vi "Configure Trigger Mode.vi"(8 "error in (no error)":errorcluster, 10 "Trigger Mode":T1, 11 "DG645 in":refnum<class "DG645.lvclass">) -> (0 "error out":errorcluster, 3 "DG645 out":refnum<class "DG645.lvclass">)   [LabVIEW 2018, in "DG645.lvlib" / "DG645.lvclass"]
uses:
  DG645.lvclass
  PPLs/Digital Delay Generator/Parent/Digital Delay Generator.lvlibp/Custom Controls/Trigger Mode.ctl
  DG645.lvclass/DG645.ctl
  <instrlib>/Stanford Research DG645/Stanford Research DG645.lvlib
  PPLs/Digital Delay Generator/Parent/Digital Delay Generator.lvlibp/Digital Delay Generator.lvclass
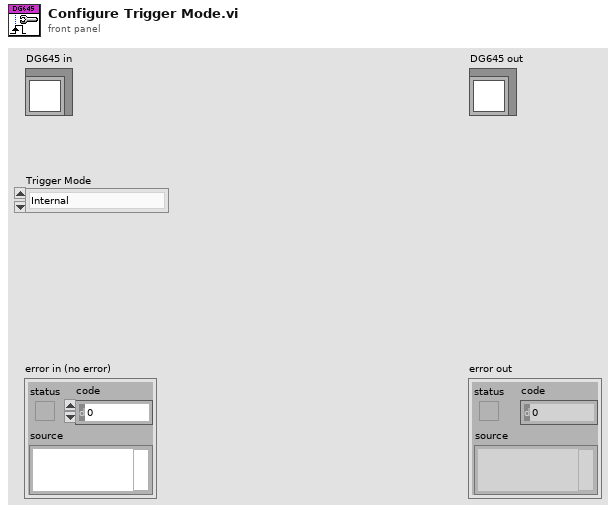
[diagram p1: front panel]
types:
  T1 = typedef "Digital Delay Generator.lvlibp/Digital Delay Generator.lvclass/Trigger Mode.ctl" = enum16{"Internal", "External Rising Edge", "External Falling Edge", "Single Shot Internal Rising Edge", "Single Shot External Rising Edge", "Single Shot", "Line"}
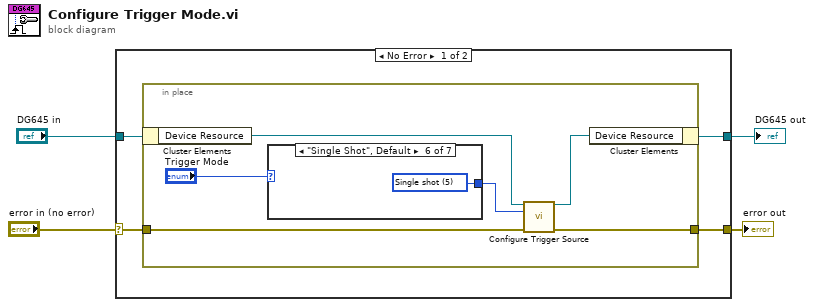
[diagram p0: block diagram]
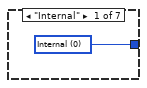
[diagram p2: hidden frame]
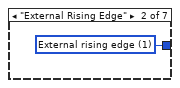
[diagram p3: hidden frame]
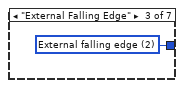
[diagram p4: hidden frame]
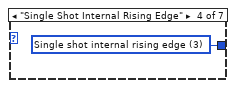
[diagram p5: hidden frame]
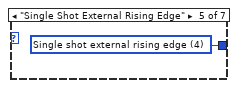
[diagram p6: hidden frame]
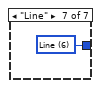
[diagram p7: hidden frame]
diagram:
  n1 = case shown="No Error" "error in (no error)" {
    selector: "error in (no error)" -> [w7 w23]
    tunnel: [w6 w23] -> w3
    tunnel: [w5 w22] -> w2
    tunnel: "DG645 in" -> [w8 w22]
    frame No Error {
      n2 = in-place {
        in-place-border: w7 -> [w13]
        in-place-border: [w12] -> w6
        n3 = in-place-cluster #1(w8) -> ("Device Resource"=w14:refnum<visa-resource-name>)
        n4 = case shown="\"Single Shot\", Default" "Trigger Mode" {
          tunnel: [w15 w16 w17 w18 w19 w20 w21] -> w10
          frame "Internal" {
            w15 = u16 0 items=["Internal", "External rising edge", "External falling edge", "Single shot internal rising edge", "Single shot external rising edge", "Single shot", "Line"] ("Trigger Source (5:Single Shot)")
          }
          frame "External Rising Edge" {
            w16 = u16 1 items=["Internal", "External rising edge", "External falling edge", "Single shot internal rising edge", "Single shot external rising edge", "Single shot", "Line"] ("Trigger Source (5:Single Shot)")
          }
          frame "External Falling Edge" {
            w17 = u16 2 items=["Internal", "External rising edge", "External falling edge", "Single shot internal rising edge", "Single shot external rising edge", "Single shot", "Line"] ("Trigger Source (5:Single Shot)")
          }
          frame "Single Shot Internal Rising Edge" {
            w18 = u16 3 items=["Internal", "External rising edge", "External falling edge", "Single shot internal rising edge", "Single shot external rising edge", "Single shot", "Line"] ("Trigger Source (5:Single Shot)")
          }
          frame "Single Shot External Rising Edge" {
            w19 = u16 4 items=["Internal", "External rising edge", "External falling edge", "Single shot internal rising edge", "Single shot external rising edge", "Single shot", "Line"] ("Trigger Source (5:Single Shot)")
          }
          frame "Single Shot", Default {
            w20 = u16 5 items=["Internal", "External rising edge", "External falling edge", "Single shot internal rising edge", "Single shot external rising edge", "Single shot", "Line"] ("Trigger Source (5:Single Shot)")
          }
          frame "Line" {
            w21 = u16 6 items=["Internal", "External rising edge", "External falling edge", "Single shot internal rising edge", "Single shot external rising edge", "Single shot", "Line"] ("Trigger Source (5:Single Shot)")
          }
        }
        n5 = call <instrlib>:"Configure Trigger Source.vi"("VISA resource name"=w14, "Trigger Source (5:Single Shot)"=w10, "error in (no error)"=w13) -> ("VISA resource name out"=w11:refnum<visa-resource-name>, "error out"=w12:errorcluster)  [unwired: 11 in]
        n6 = in-place-cluster #1("Device Resource"=w11) -> (w5:refnum<class "DG645.lvclass">)
      }
    }
    frame Error {
    }
  }
  "error out" <- w3
  "DG645 out" <- w2
